vi "CANbus config to JSON.vi"(8 "error in":errorcluster) -> (0 "error out":errorcluster, 3 "<JSON>":string)   [LabVIEW 2021]
uses:
  48ea5a33-1648-4ef8-86a8-e898ef81ae33.vi
  <vilib>/JDP Science/JSONtext/Variant to JSON Text.vi
  <vilib>/JDP Science/JSONtext/LVClass Serializer/JSONtext LVClass Serializer.lvclass
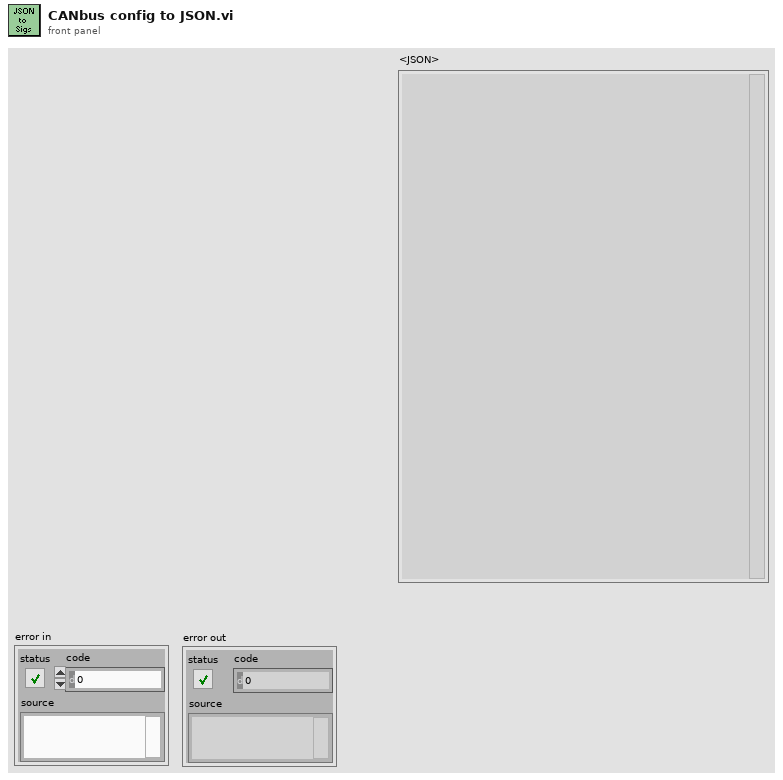
[diagram p1: front panel]
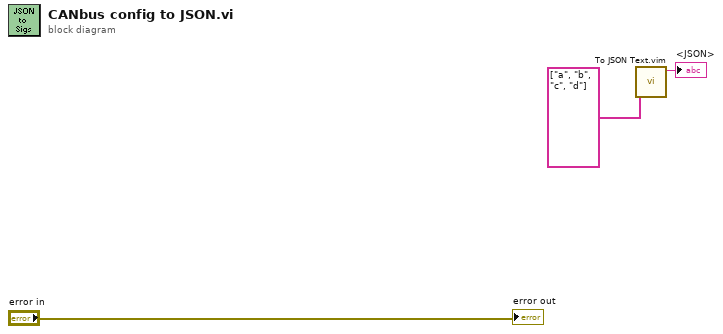
[diagram p0: block diagram]
diagram:
  n1 = call "To JSON Text.vim"("Anything"=string[] ["a", "b", "c", "d"]) -> ("<JSON>"=→"<JSON>":string)  [unwired: 9 in, 1 out]
  "error out" <- "error in"
